vi "sample_arduino.vi"() -> ()   [LabVIEW 2016]
uses:
  <vilib>/Instr/_visa.llb/VISA Configure Serial Port (Instr).vi
panel:
  out "read buffer":string
  in  "stop":bool
  in  "VISA resource name":refnum<visa-resource-name>
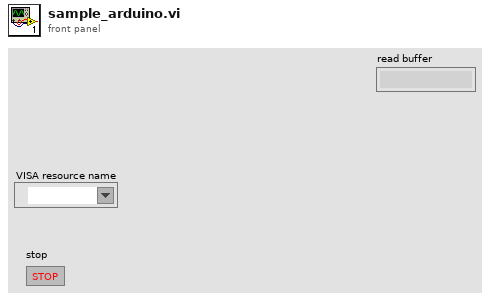
[diagram p1: front panel]
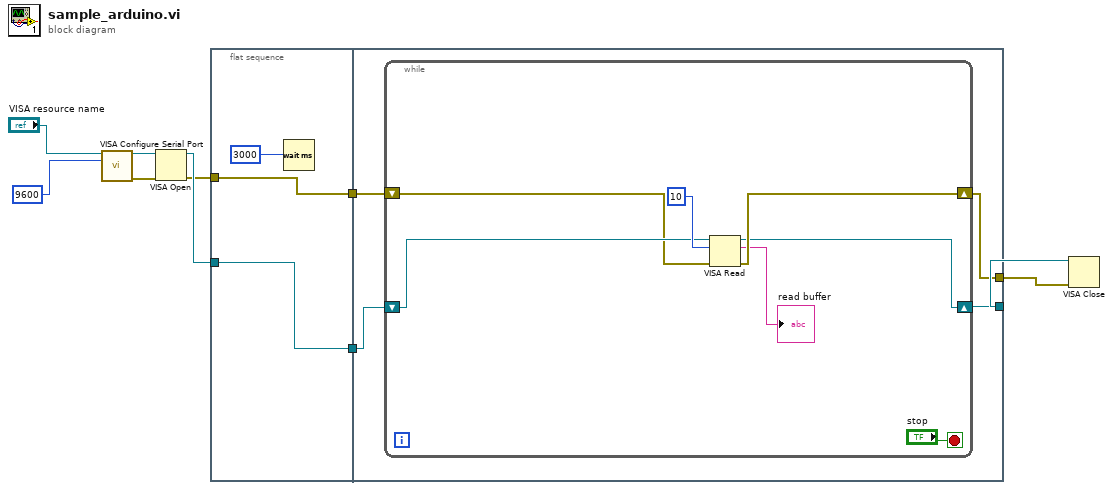
[diagram p0: block diagram]
diagram:
  n1 = call-poly "VISA Configure Serial Port"("VISA resource name"="VISA resource name", "baud rate (9600)"=9600) -> ("VISA resource name out"=w8:refnum<visa-resource-name>, "error out"=w7:errorcluster)  [unwired: 12 in]
  n2 = VISA Open(error in (no error)=w7, VISA resource name=w8) -> (VISA resource name=w5:refnum<visa-resource-name>, error out=w2:errorcluster)  [unwired: 3 in]
  n3 = flat-sequence {
    tunnel: [w12] -> w6
    tunnel: w5 -> [w12]
    tunnel: [w11] -> w3
    tunnel: w2 -> [w11]
    tunnel: w6 -> [w17]
    tunnel: [w16] -> w4
    tunnel: w3 -> [w15]
    tunnel: [w14] -> w1
    frame #0 {
      n4 = Wait (ms)(milliseconds to wait=3000) -> ()  [unwired: 1 out]
    }
    frame #1 {
      n5 = while {
        shift-right: [w22] -> w16
        shift-left: w17 -> [w20]
        shift-right: [w23] -> w14
        shift-left: w15 -> [w19]
        stop <- "stop" stop-if-true
        n6 = VISA Read(VISA resource name=w20, byte count=10, error in (no error)=w19) -> (VISA resource name out=w22:refnum<visa-resource-name>, read buffer=→"read buffer":string, error out=w23:errorcluster)  [unwired: 1 out]
      }
    }
  }
  n7 = VISA Close(VISA resource name=w4, error in (no error)=w1) -> ()  [unwired: 1 out]
